vi "CreateLogCSVString.vi"(8 "Error In":errorcluster, 11 "Log Data":T1[](array[typedef])) -> (0 "Error Out":errorcluster, 3 "CSV String":string)   [LabVIEW 2012]
uses:
  HardwareLogData.ctl
  HardwareDisplayData.ctl
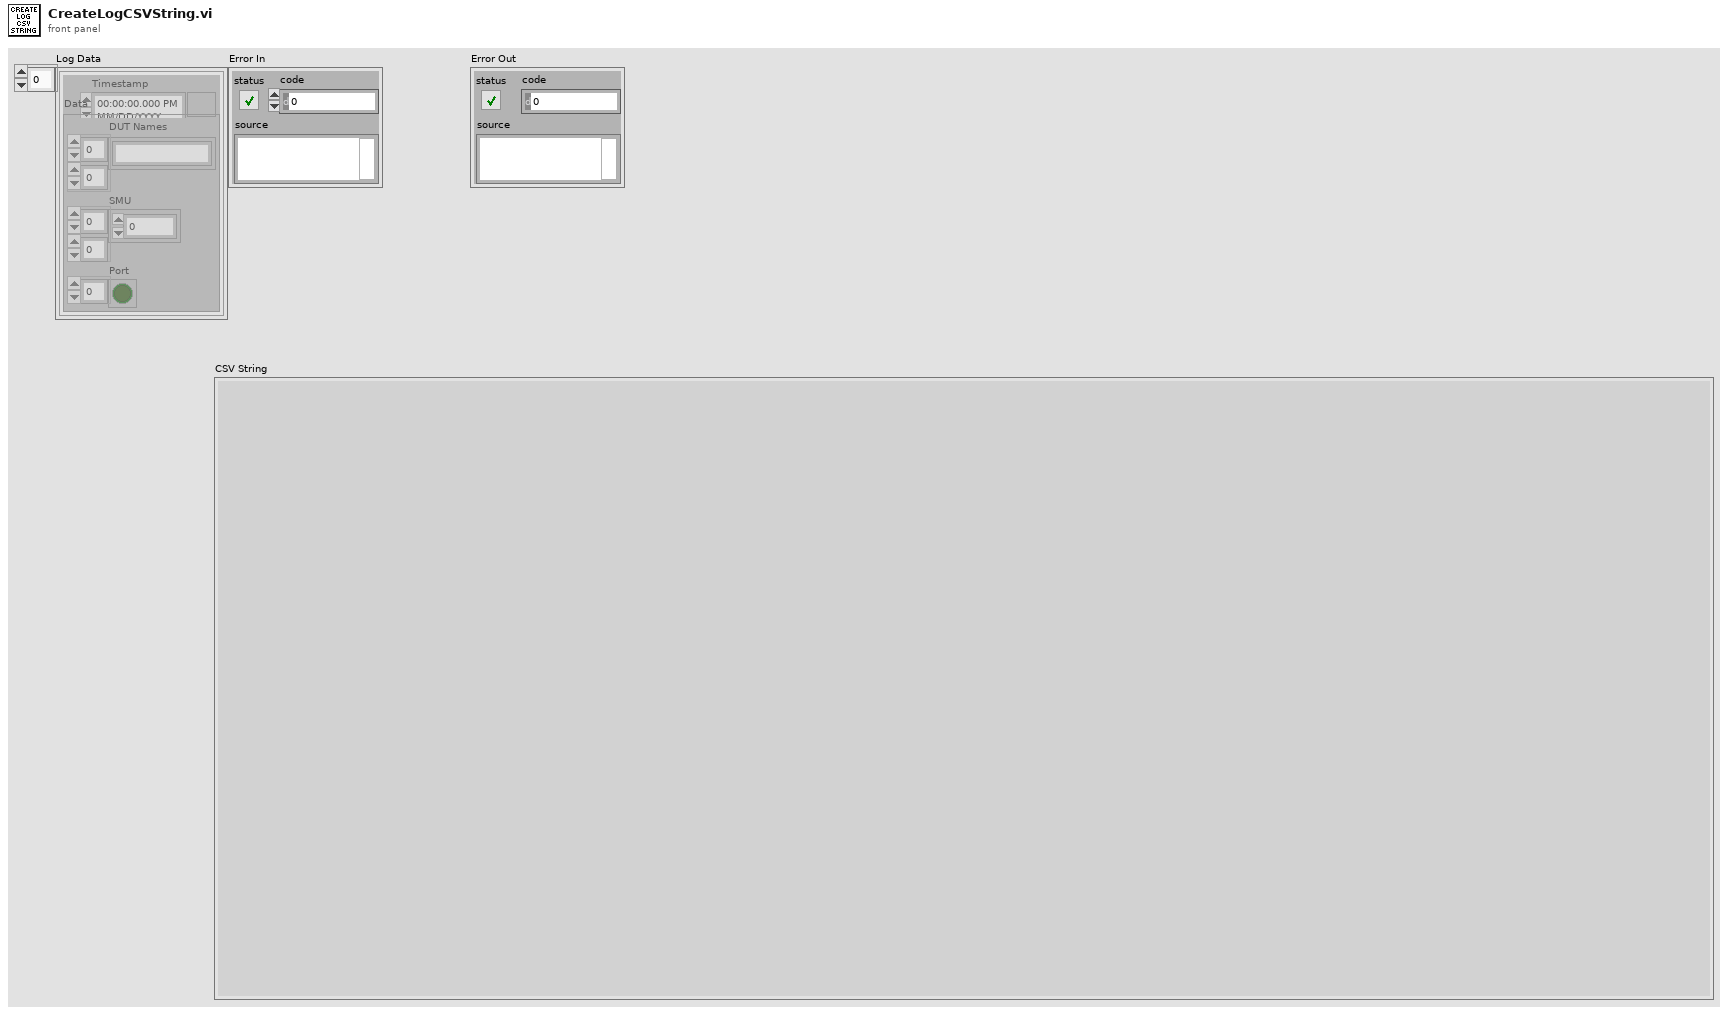
[diagram p1: front panel]
types:
  T1 = typedef "HardwareLogData.ctl" = cluster{"Timestamp":timestamp, "Data":T2}
  T2 = typedef "HardwareDisplayData.ctl" = cluster{"DUT Names":string[][], "SMU":dbl[][], "Port":bool[]}
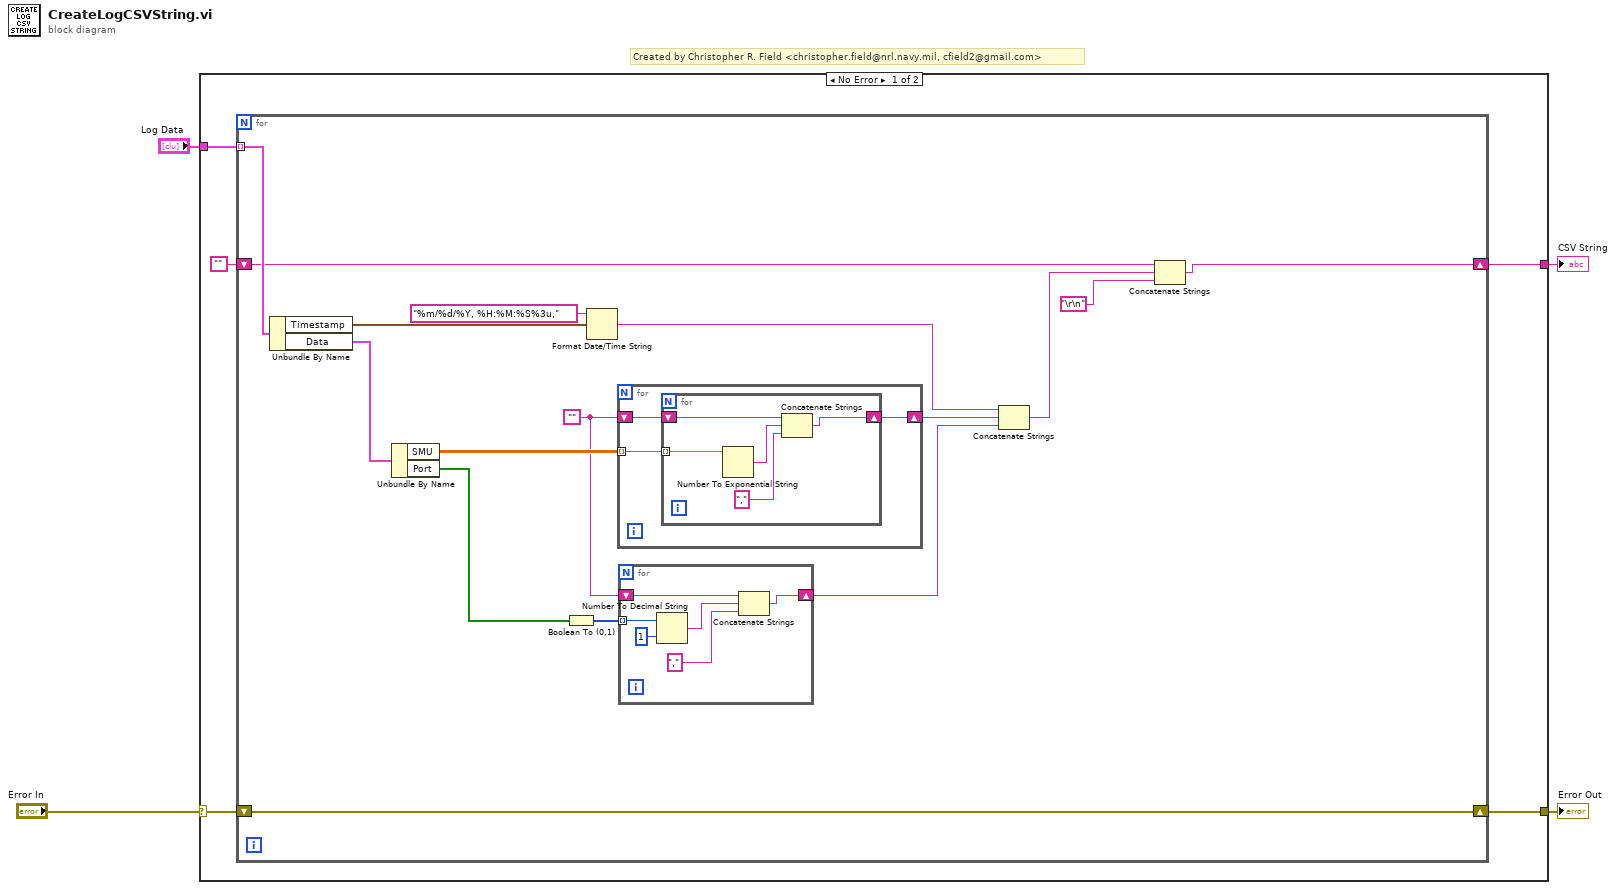
[diagram p0: block diagram]
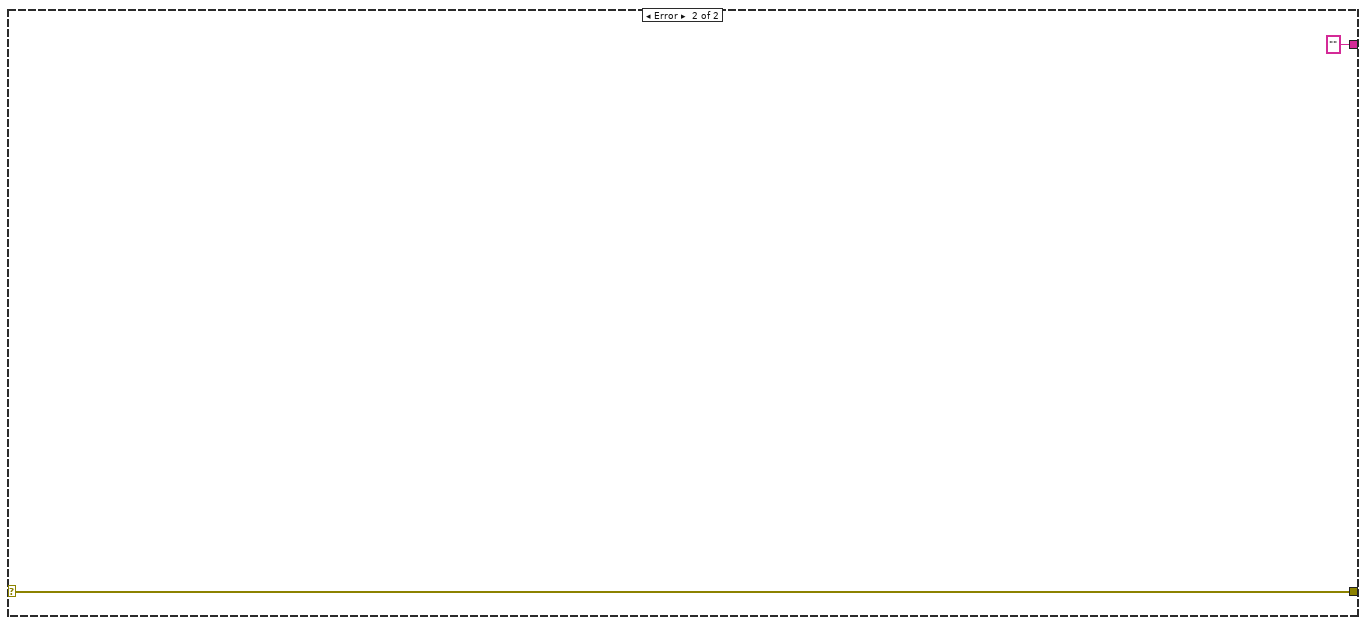
[diagram p2: hidden frame]
diagram:
  # "Created by Christopher R. Field <christopher.field@nrl.navy.mil, cfield2@gmail.com>"
  n1 = case shown="No Error" "Error In" {
    selector: "Error In" -> [w8 w41]
    tunnel: "Log Data" -> [w9 _]
    tunnel: [w7 w41] -> w2
    tunnel: [w5 ""] -> w1
    frame No Error {
      n2 = for {
        tunnel: w9 -> [w24] mode=indexing
        shift-right: [w25] -> w7
        shift-left: w8 -> [w25]
        shift-right: [w10] -> w5
        shift-left: "" -> [w13]
        w17 = ""
        n3 = Unbundle By Name(w24) -> ("Timestamp"=w22:timestamp, "Data"=w23:T2)
        n4 = Unbundle By Name(w23) -> ("SMU"=w20:dbl[][], "Port"=w19:bool[])
        n5 = Boolean To (0,1)(Boolean=w19) -> (0, 1=w18:i16[])
        n6 = Format Date/Time String(time format string (%c)="%m/%d/%Y, %H:%M:%S%3u,", seconds (now)=w22) -> (date/time string=w14:string)  [unwired: 1 in]
        n7 = for {
          tunnel: w20 -> [w34] mode=indexing
          shift-right: [w32] -> w16
          shift-left: w17 -> [w33]
          n8 = for {
            tunnel: w34 -> [w39] mode=indexing
            shift-right: [w35] -> w32
            shift-left: w33 -> [w38]
            n9 = Number To Exponential String(number=w39) -> (E-format string=w37:string)  [unwired: 3 in]
            n10 = Concatenate Strings(w38, w37, "," ("string")) -> (w35:string)
          }
        }
        n11 = for {
          tunnel: w18 -> [w30] mode=indexing
          shift-right: [w26] -> w15
          shift-left: w17 -> [w31]
          n12 = Number To Decimal String(number=w30, width (-)=i16 1) -> (decimal integer string=w28:string)
          n13 = Concatenate Strings(w31, w28, "," ("string")) -> (w26:string)
        }
        n14 = Concatenate Strings(w14, w16, w15) -> (w12:string)
        n15 = Concatenate Strings(w13, w12, "\r\n") -> (w10:string)
      }
    }
    frame Error {
    }
  }
  "Error Out" <- w2
  "CSV String" <- w1
